vi "Hardware Device Get Info.vi"(8 "error in":errorcluster, 11 "NI PWM Input in":refnum<class "NI PWM Input.lvclass">) -> (0 "error out":errorcluster, 3 "NI PWM Input out":refnum<class "NI PWM Input.lvclass">)   [LabVIEW 2023, in "HardwareAbstractionLayer_LVOOP.lvlib" / "NI PWM Input.lvclass"]
doc: "This VI is AI Physical Channel Read"
uses:
  NI PWM Input.lvclass
  NI PWM Input.lvclass/NI PWM Input.ctl
  <resource>/objmgr/daqmx.rc
  Teststand/Teststand.lvclass
panel:
  out "CI.PhysicalChans":tag[](array[tag])
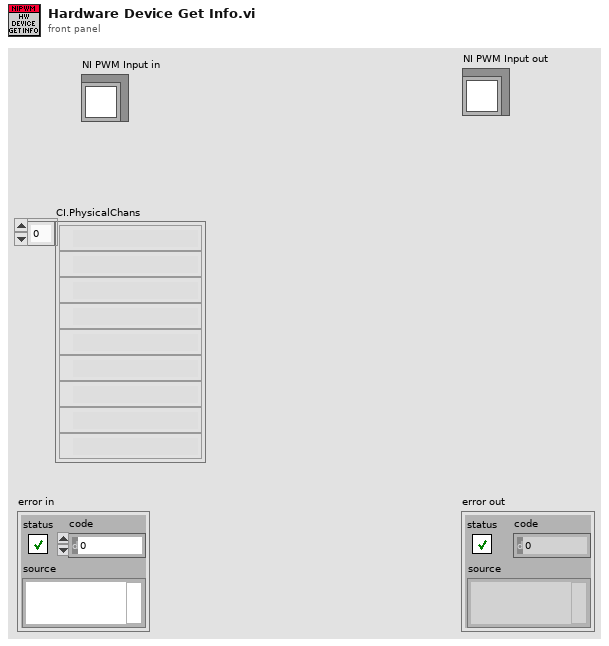
[diagram p1: front panel]
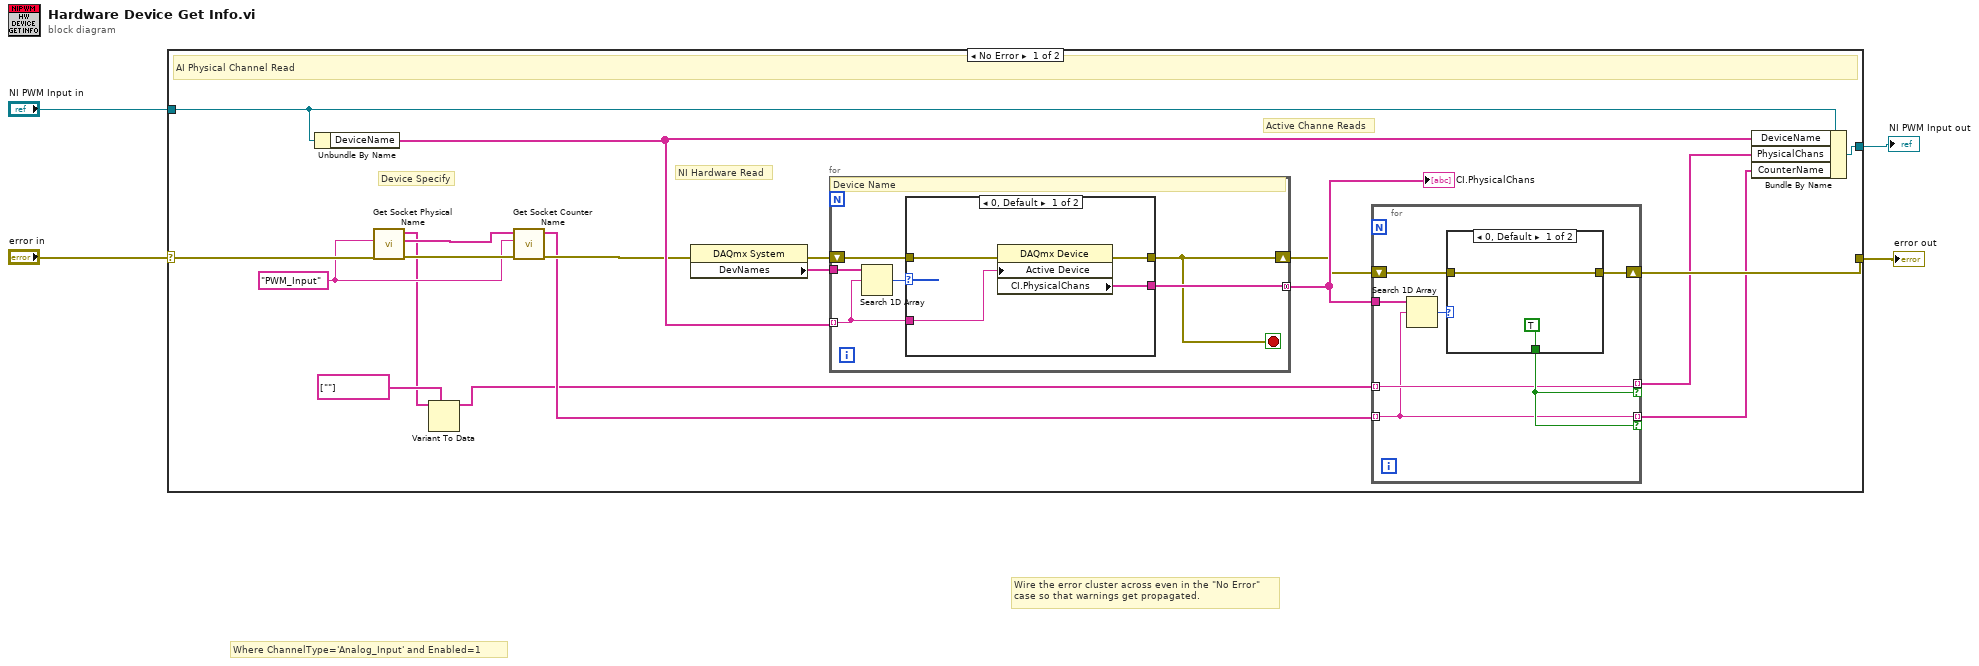
[diagram p0: block diagram]
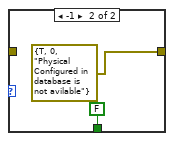
[diagram p2: hidden frame]
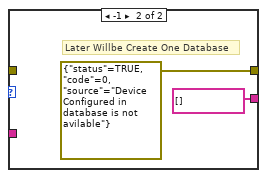
[diagram p3: hidden frame]
diagram:
  # "Where ChannelType='Analog_Input' and Enabled=1"
  # "Wire the error cluster across even in the \"No Error\"\ncase so that warnings get propagated."
  n1 = case shown="No Error" "error in" {
    selector: "error in" -> [w14 w48]
    tunnel: [w16 w48] -> w3
    tunnel: [w23 w47] -> w1
    tunnel: "NI PWM Input in" -> [w22 w47]
    frame No Error {
      w10 = "PWM_Input" ("ChannelType")
      # "Active Channe Reads"
      # "Device Specify"
      # "NI Hardware Read"
      # "AI Physical Channel Read"
      n2 = Unbundle By Name(w22) -> ("DeviceName"=w21:tag[])
      n3 = call "Get Socket Physical Name.vi"("error In"=w14, "ChannelType"=w10) -> ("error out"=w13:errorcluster, "Physical Channel"=w11:tag[], "Physical String"=w6:string[])  [unwired: 7 in]
      n4 = Variant To Data(type=tag[] [""], Variant=w6) -> (data=w5:tag[])  [unwired: 1 in, 1 out]
      n5 = call "Get Socket Counter Name.vi"("error In"=w13, "ChannelType"=w10, "Physical Channel"=w11) -> ("error out"=w12:errorcluster, "CounterName"=w9:tag[])  [unwired: 6 in, 1 out]
      n6 = property class="DAQmx System"(error in=w12) -> (error out=w19:errorcluster, "DevNames"=w20:tag[])  [unwired: 1 in, 1 out]
      n7 = for {
        tunnel: w21 -> [w37] mode=indexing
        tunnel: w20 -> [w38]
        tunnel: [w36] -> w18 mode=concatenating
        shift-right: [w35] -> w17
        shift-left: w19 -> [w39]
        stop <- w35 stop-if-true
        # "Device Name"
        n8 = Search 1D Array(1D array=w38, element=w37) -> (index of element=w40:i32)  [unwired: 1 in]
        n9 = case shown="0, Default" w40 {
          tunnel: w39 -> [w42 _]
          tunnel: [w41 errorcluster {"status"=TRUE, "code"=0, "source"="Device  Configured in database is not avilable"} ("error out")] -> w35
          tunnel: w37 -> [w44 _]
          tunnel: [w43 tag[] [] ("AI.PhysicalChans")] -> w36
          frame 0, Default {
            n10 = property class="DAQmx Device"(error in=w42, "Active Device"=w44) -> (error out=w41:errorcluster, "CI.PhysicalChans"=w43:tag[])  [unwired: 1 in, 1 out]
          }
          frame -1 {
            # "Later Willbe Create One Database"
          }
        }
      }
      "CI.PhysicalChans" <- w18
      n11 = for {
        tunnel: w18 -> [w30]
        tunnel: w5 -> [w25] mode=indexing
        shift-right: [w27] -> w16
        shift-left: w17 -> [w28]
        tunnel: [w25] -> w15 mode=indexing if=w26
        tunnel: w9 -> [w24] mode=indexing
        tunnel: [w24] -> w8 mode=indexing if=w26
        n12 = Search 1D Array(1D array=w30, element=w24) -> (index of element=w29:i32)  [unwired: 1 in]
        n13 = case shown="0, Default" w29 {
          tunnel: w28 -> [w32 _]
          tunnel: [w32 errorcluster {"status"=TRUE, "code"=0, "source"="Physical Configured in database is not avilable"} ("error out")] -> w27
          tunnel: [TRUE FALSE] -> w26
          frame 0, Default {
          }
          frame -1 {
          }
        }
      }
      n14 = Bundle By Name(cluster=w22, "DeviceName"=w21, "PhysicalChans"=w15, "CounterName"=w8) -> (w23:refnum<class "NI PWM Input.lvclass">)
    }
    frame Error {
    }
  }
  "error out" <- w3
  "NI PWM Input out" <- w1
